vi "w8_Event_Example.vi"() -> ()   [LabVIEW 2020]
uses:
  <vilib>/Utility/miscctls.llb/LVPoint32TypeDef.ctl
panel:
  in  "String":string
  in  "color(black)":u32(colorbox)
  out "2D Picture":picture
  out "Numeric":i32
  out "Coords":T1
  in  "Slide":dbl(slide) scale=0.0..10.0
  in  "stop":bool
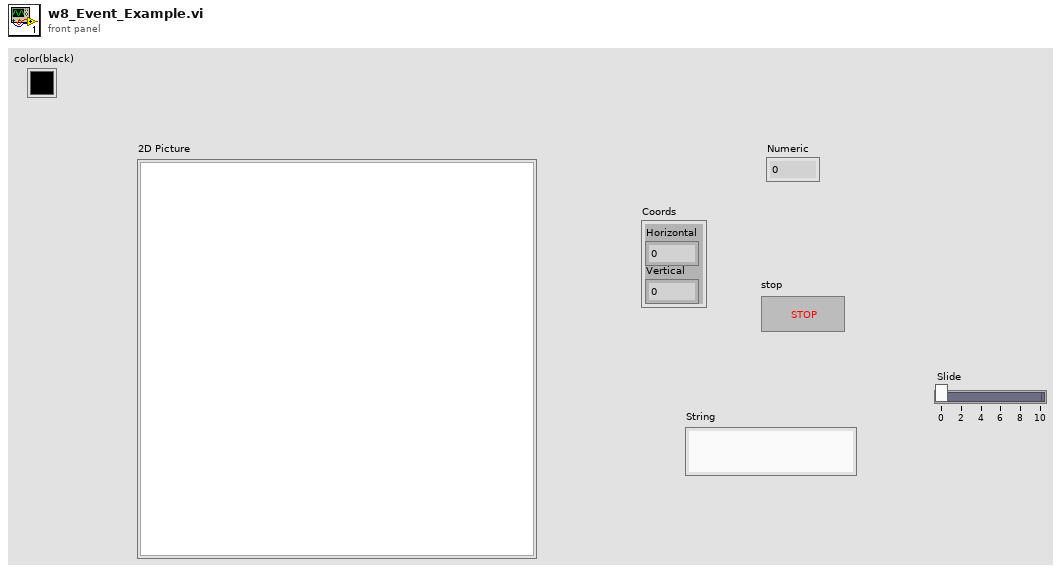
[diagram p1: front panel]
types:
  T1 = typedef "LVPoint32TypeDef.ctl" = cluster{"Horizontal":i32, "Vertical":i32}
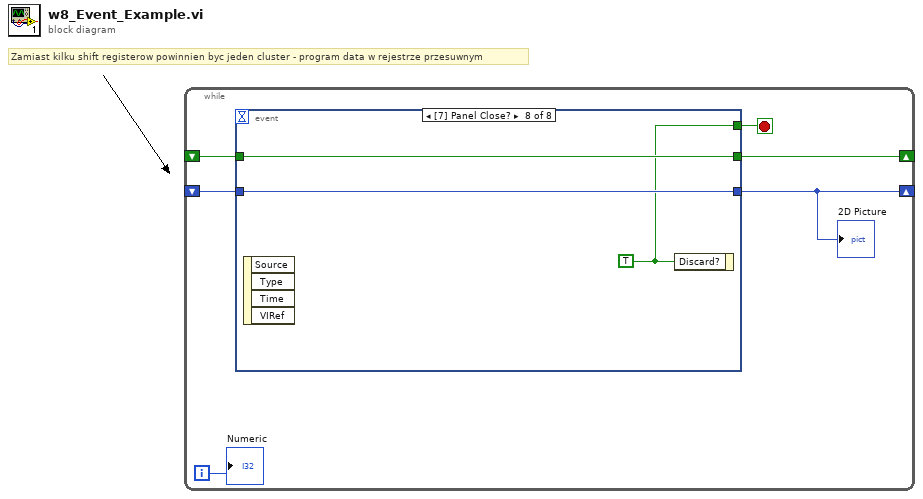
[diagram p0: block diagram]
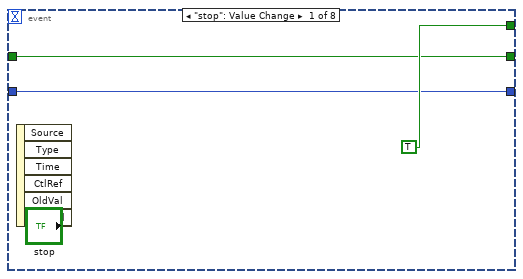
[diagram p2: hidden frame]
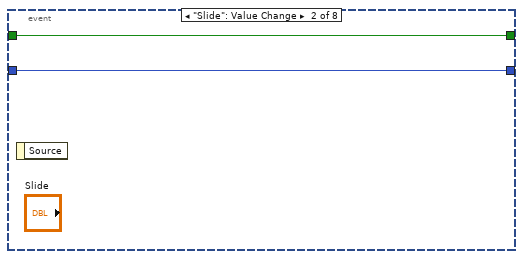
[diagram p3: hidden frame]
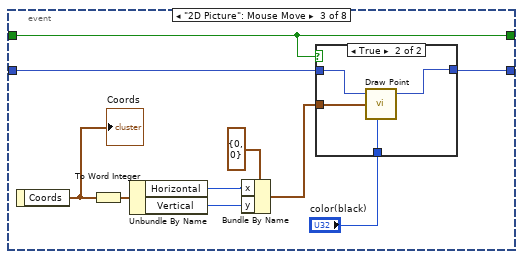
[diagram p4: hidden frame]
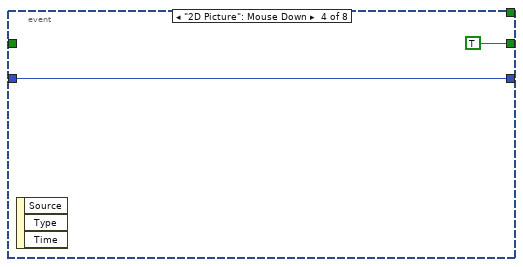
[diagram p6: hidden frame]
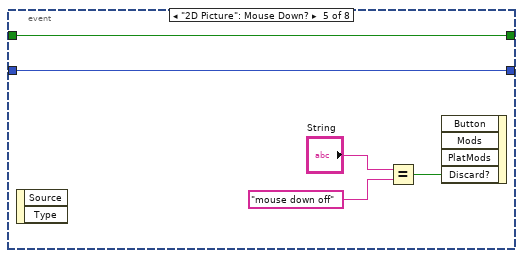
[diagram p7: hidden frame]
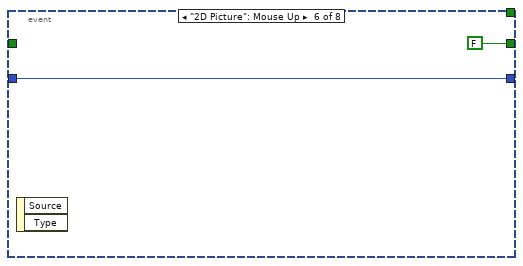
[diagram p8: hidden frame]
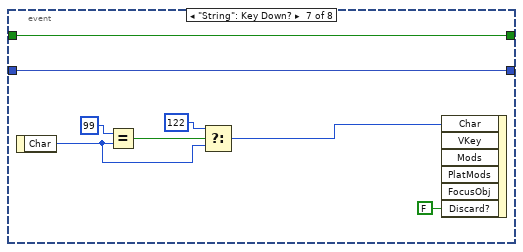
[diagram p9: hidden frame]
diagram:
  # "Zamiast kilku shift registerow powinnien byc jeden cluster - program data w rejestrze przesuwnym"
  n1 = while {
    shift-right: [w1] -> _
    shift-left: _ -> [w4]
    shift-right: [w3] -> _
    shift-left: _ -> [w2]
    i -> [w5]
    stop <- w6 stop-if-true
    n2 = event shown="[7] Panel Close?" {
      selector: _ -> [_ _ _ _ _ _ _ _]
      dyn-events: _ -> [_ _ _ _ _ _ _ _]
      timeout: _ -> [_ _ _ _ _ _ _ _]
      tunnel: [TRUE ("stop") _ _ _ _ _ _ w44] -> w6
      tunnel: [w8 w11 w14 w28 w33 w35 w43 w46] -> w1
      tunnel: w4 -> [w8 w11 w15 w28 w33 w35 w43 w46]
      tunnel: [w7 w10 w13 TRUE w29 FALSE w42 w45] -> w3
      tunnel: w2 -> [w7 w10 w13 _ w29 _ w42 w45]
      event "stop": Value Change {
        n3 = event-data() -> ()  [unwired: 1 in, 6 out]
      }
      event "Slide": Value Change {
        n4 = event-data() -> ()  [unwired: 1 in, 1 out]
      }
      event "2D Picture": Mouse Move {
        n5 = event-data() -> ("Coords"=w21:T1)  [unwired: 1 in]
        "Coords" <- w21
        n6 = To Word Integer(number=w21) -> (16bit integer=w17:cluster{"Horizontal":i16, "Vertical":i16})
        n7 = Unbundle By Name(w17) -> ("Horizontal"=w18:i16, "Vertical"=w19:i16)
        n8 = Bundle By Name(cluster=cluster{"x":i16, "y":i16} {"x"=0, "y"=0} ("point(x,y)"), "x"=w18, "y"=w19) -> (w16:cluster{"x":i16, "y":i16})
        n9 = case shown="True" w13 {
          tunnel: w16 -> [_ w26]
          tunnel: w15 -> [w22 w25]
          tunnel: [w22 w24] -> w14
          tunnel: "color(black)" -> [_ w23]
          frame False {
          }
          frame True {
            n10 = call <vilib>:"Draw Point.vi"("picture"=w25, "point(x,y)"=w26, "color(black)"=w23) -> ("new picture"=w24:picture)  [unwired: 6 in]
          }
        }
      }
      event "2D Picture": Mouse Down {
        n11 = event-data() -> ()  [unwired: 1 in, 3 out]
      }
      event "2D Picture": Mouse Down? {
        n12 = event-data() -> ()  [unwired: 1 in, 2 out]
        n13 = Equal?(x="String", y="mouse down off" ("String")) -> (x = y?=w30:bool)
        n14 = event-data("Discard?"=w30) -> ()  [unwired: 4 in, 1 out]
      }
      event "2D Picture": Mouse Up {
        n15 = event-data() -> ()  [unwired: 1 in, 2 out]
      }
      event "String": Key Down? {
        n16 = event-data() -> ("Char"=w39:i16)  [unwired: 1 in]
        n17 = Equal?(x=i16 99, y=w39) -> (x = y?=w41:bool)
        n18 = Select(t=i16 122, s=w41, f=w39) -> (s? t:f=w37:i16)
        n19 = event-data("Char"=w37, "Discard?"=FALSE) -> ()  [unwired: 5 in, 1 out]
      }
      event Panel Close? {
        w44 = TRUE ("Discard?")
        n20 = event-data() -> ()  [unwired: 1 in, 4 out]
        n21 = event-data("Discard?"=w44) -> ()  [unwired: 1 in, 1 out]
      }
    }
    "2D Picture" <- w1
    "Numeric" <- w5
  }
